vi "Main.vi"() -> ()   [LabVIEW 2019]
uses:
  <vilib>/MakerHub/LINX/Public/Utilities/Open Local.vi
  Demo 2 Sensor_SHT21/SHT21_class/SHT21.lvclass
  <vilib>/MakerHub/LINX/LMH-LINX.lvlib
  WebServiceData_class/WebServiceData.lvclass
panel:
  out "output cluster":cluster{"T":dbl, "RH":dbl}
  in  "stop":bool
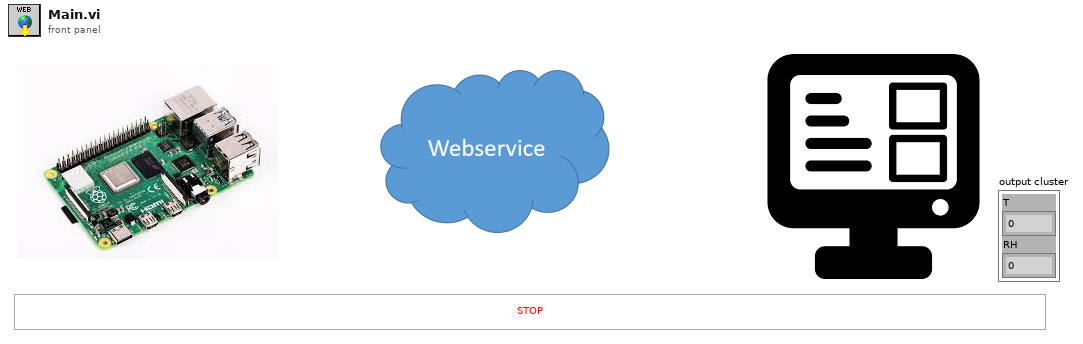
[diagram p1: front panel]
types:
  T1 = typedef "LMH-LINX.lvlib/LINX Ref.ctl" = cluster{"IO":T2, "Interface":T3, "LINX Device Config":T4}
  T2 = typedef "LMH-LINX.lvlib/Platform.ctl" = enum16{"Remote", "Local"}
  T3 = typedef "LMH-LINX.lvlib/Interface.ctl" = enum16{"Serial", "TCP"}
  T4 = typedef "LMH-LINX.lvlib/Device.lvlib/LINX Device Config.ctl" = cluster{"Interface":T3, "COM Port":refnum<visa-resource-name>, "TCP Configuration":T5, "Device Family":u8, "Device ID":u8, "Device Name":string, "TCP Ref":refnum<k5>, "Channels":T6}
  T5 = typedef "LMH-LINX.lvlib/Device.lvlib/TCP Config.ctl" = cluster{"IP Address":string, "Port":u16}
  T6 = typedef "LMH-LINX.lvlib/Channels.ctl" = cluster{"DI":u8[], "DO":u8[], "AI":u8[], "AO":u8[], "PWM":u8[], "QE":u8[], "UART":u8[], "I2C 2":u8[], "SPI":u8[], "CAN":u8[], "Servo":u8[], "AI Ref (V)":dbl, "AI Resolution (Bits)":u8, "AO Ref (V)":dbl, "AO Resolution (Bits)":u8}
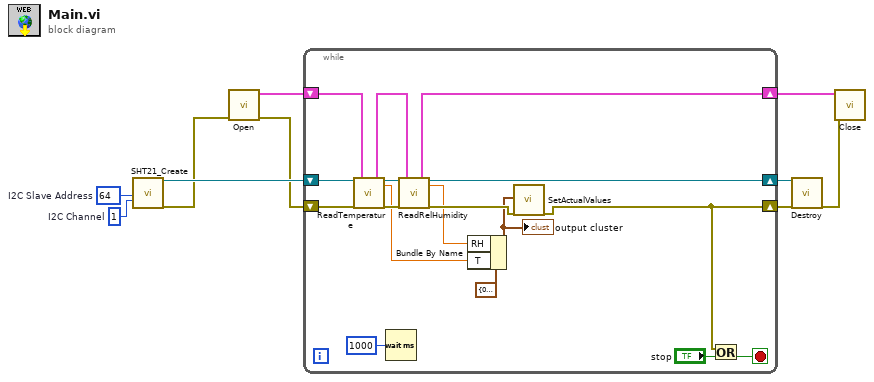
[diagram p0: block diagram]
diagram:
  w2 = u8 1  # I2C Channel
  w8 = u8 64  # I2C Slave Address
  n1 = call "SHT21_Create.vi"("I2C Slave Address (0)"=w8, "I2C Channel (0)"=w2) -> ("reference out"=w6:refnum<class "SHT21.lvclass">, "error out"=w1:errorcluster)  [unwired: 16 in]
  n2 = call-poly <vilib>:"Open.vi"("Error In"=w1) -> ("Error Out"=w3:errorcluster, "LINX Resource"=w4:T1)  [unwired: 8 in, 1 out]
  n3 = while {
    shift-right: [w19] -> w10
    shift-left: w6 -> [w23]
    shift-right: [w14] -> w9
    shift-left: w3 -> [w15]
    shift-right: [w17] -> w7
    shift-left: w4 -> [w22]
    stop <- w24 stop-if-true
    n4 = call-dynamic "ReadTemperature.vi"("reference in"=w23, "LINX Resource"=w22) -> ("LINX Resource"=w18:T1, "reference out"=w20:refnum<class "SHT21.lvclass">, "Temperature"=w11:dbl)  [unwired: 13 in, 2 out]
    n5 = Wait (ms)(milliseconds to wait=u32 1000) -> ()  [unwired: 1 out]
    n6 = call-dynamic "ReadRelHumidity.vi"("reference in"=w20, "LINX Resource"=w18) -> ("LINX Resource"=w17:T1, "reference out"=w19:refnum<class "SHT21.lvclass">, "RH"=w12:dbl)  [unwired: 13 in, 2 out]
    n7 = Bundle By Name(cluster=cluster{"T":dbl, "RH":dbl} {"T"=0.0, "RH"=0.0} ("ActualValues"), "RH"=w12, "T"=w11) -> (w13:cluster{"T":dbl, "RH":dbl})
    "output cluster" <- w13
    n8 = call "SetActualValues.vi"("ActualValues"=w13, "error in (no error)"=w15) -> ("error out"=w14:errorcluster)  [unwired: 17 in]
    n9 = Or(x=w14, y="stop") -> (x .or. y?=w24:bool)
  }
  n10 = call-dynamic "Destroy.vi"("reference in"=w10, "error in (no error)"=w9) -> ("error out"=w5:errorcluster)  [unwired: 16 in, 1 out]
  n11 = call <vilib>:"Close.vi"("Error In"=w5, "LINX Resource"=w7) -> ()  [unwired: 9 in, 1 out]
